vi "Example3.vi"   [LabVIEW 2016]
uses:
  <vilib>/NXT/Block Support/NXT_InputPort.ctl
  <vilib>/NXT/Hardware/Plugins/Tetrix DC Motor/TetrixDCMotorAddress.ctl
  <vilib>/NXT/NXTIO Xnodes/NXTIONodeSubVIs/TETRIX IO Move DC Motors.vi
  <vilib>/NXT/Dual Mode Library/Waits/Wait_EV3_Angle_Less.vi
  <vilib>/NXT/NXTIO Xnodes/NXTIONodeSubVIs/TETRIX IO Stop DC Motors.vi
  <vilib>/NXT/Dual Mode Library/Waits/Wait_Num.vi
  <vilib>/NXT/Dual Mode Library/Waits/Wait_EV3_Angle_Greater.vi
  <vilib>/NXT/Subs/LVHSConnector.ctl
  <vilib>/NXT/NXTIO Xnodes/AddressXNode/NXTIOAddress.xnode
  Test.lvrbt
  <vilib>/NXT/NXTIO Xnodes/NXTIOXNode/NXTIO.xnode
  <vilib>/NXT/LegoClasses/BrickReference/BrickReference.lvclass
types:
  T1 = typedef "NXT_InputPort.ctl" = u32
  T2 = typedef "TetrixDCMotorAddress.ctl" = i32
  T3 = typedef "LVHSConnector.ctl" = refnum<class "BrickReference.lvclass">
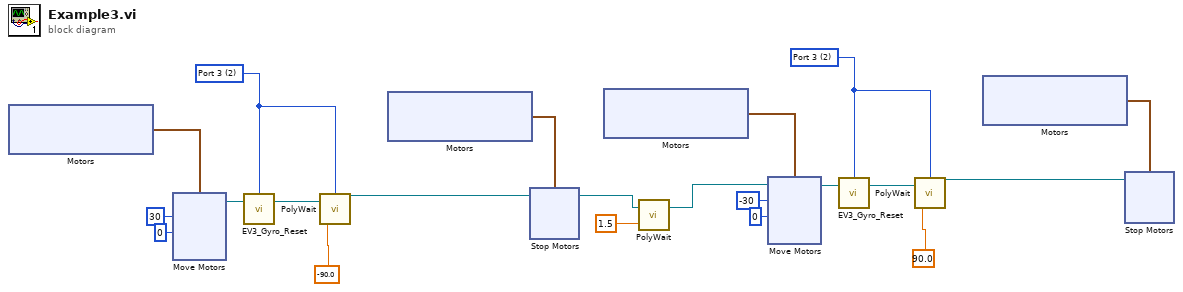
[diagram p0: block diagram]
diagram:
  w10 = T1 2 items=["Port 1", "Port 2", "Port 3", "Port 4"] ("Port (Port 1)")
  w15 = T1 2 items=["Port 1", "Port 2", "Port 3", "Port 4"] ("Port (Port 1)")
  n1 = xnode "Motors"() -> ("Motor"=w21:cluster{"TetrixDCMotor":T2, "TetrixDCMotor":T2})
  n2 = xnode "Move Motors"("Power/Speed 2"=i8 0, "Power/Speed 1"=i8 30, "Motors"=w21) -> ("NXT/EV3"=w17:T3)  [unwired: 1 in]
  n3 = call <vilib>:"EV3_Gyro_Reset.vi"("NXT/EV3"=w17, "Port (Port 1)"=w15) -> ("NXT/EV3"=w16:T3)  [unwired: 2 in]
  n4 = call-poly <vilib>:"PolyWait.vi"("Degrees (180)"=sgl -90.0, "NXT/EV3"=w16, "Port (Port 1)"=w15) -> ("NXT/EV3"=w14:T3)  [unwired: 1 in]
  n5 = xnode "Motors"() -> ("Motor"=w18:cluster{"TetrixDCMotor":T2, "TetrixDCMotor":T2})
  n6 = xnode "Stop Motors"("Motors"=w18, "NXT/EV3"=w14) -> ("NXT/EV3"=w3:T3)
  n7 = xnode "Motors"() -> ("Motor"=w4:cluster{"TetrixDCMotor":T2, "TetrixDCMotor":T2})
  n8 = call-poly <vilib>:"PolyWait.vi"("Time (1 sec)"=sgl 1.5, "NXT/EV3"=w3) -> ("NXT/EV3"=w2:T3)  [unwired: 2 in]
  n9 = xnode "Move Motors"("Power/Speed 2"=i8 0, "Power/Speed 1"=i8 -30, "Motors"=w4, "NXT/EV3"=w2) -> ("NXT/EV3"=w8:T3)
  n10 = call <vilib>:"EV3_Gyro_Reset.vi"("NXT/EV3"=w8, "Port (Port 1)"=w10) -> ("NXT/EV3"=w9:T3)  [unwired: 2 in]
  n11 = call-poly <vilib>:"PolyWait.vi"("Degrees (180)"=sgl 90.0, "NXT/EV3"=w9, "Port (Port 1)"=w10) -> ("NXT/EV3"=w11:T3)  [unwired: 1 in]
  n12 = xnode "Motors"() -> ("Motor"=w7:cluster{"TetrixDCMotor":T2, "TetrixDCMotor":T2})
  n13 = xnode "Stop Motors"("Motors"=w7, "NXT/EV3"=w11) -> ()  [unwired: 1 out]
